vi "Fix Format String on Representation Change.vi"(8 "error in (no error)":errorcluster, 11 "Numeric Data Type in":refnum<class "Numeric Data Type.lvclass">) -> (0 "error out":errorcluster, 3 "Numeric Data Type out":refnum<class "Numeric Data Type.lvclass">)   [LabVIEW 2018, in "Numeric Data Type.lvclass"]
uses:
  Numeric Data Type.lvclass
  Numeric Data Type.lvclass/Numeric Data Type.ctl
  Numeric Format Enum.ctl
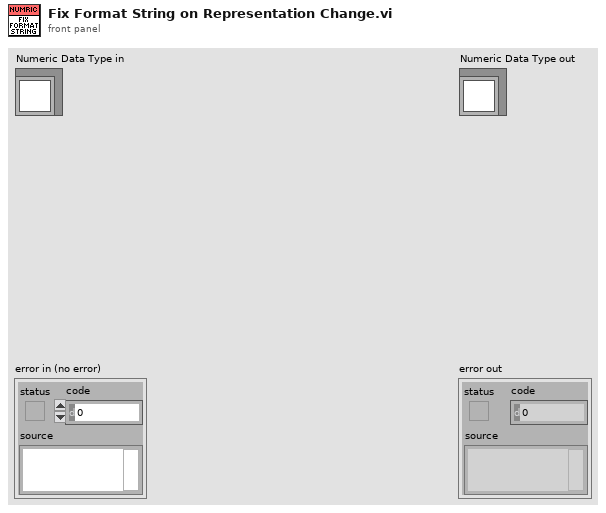
[diagram p1: front panel]
types:
  T1 = typedef "Numeric Data Type.lvclass/Numeric Format Enum.ctl" = enum16{"Floating Point Notation", "Scientific Notation", "Engineering Notation", "SI Notation", "<not used>", "Decimal", "Hexadecimal", "Octal", "Binary", "<not used 2>", "Absolute Time", "Relative Time"}
  T2 = typedef "Numeric Data Type.lvclass/Representation Enum.ctl" = enum16{"Extended (EXT)", "Double (DBL)", "Single (SGL)", "Fixed-Point (FXP)", "Quad Integer (I64)", "Long Integer (I32)", "Word Integer (I16)", "Byte Integer (I8)", "Unsigned Quad (U64)", "Unsigned Long (U32)", "Unsigned Word (U16)", "Unsigned Byte (U8)", "Complex Extended (CXT)", "Complex Double (CDB)", "Complex Single (CSG)"}
  T3 = typedef "Numeric Data Type.lvclass/Numeric Info.ctl" = cluster{"Minimum Field Width":i32, "Digits of Precision":i32, "Numeric Format":T1, "Precision Type":T4, "Hide trailing zeros":bool, "exponent":bool, "just/pad":T5, "Modifiers":string}
  T4 = typedef "Numeric Data Type.lvclass/Precision Type.ctl" = enum16{"Digits of precision", "Significant digits"}
  T5 = typedef "Numeric Data Type.lvclass/Padding.ctl" = enum16{"Pad with spaces on left", "Pad with spaces on right", "Pad with zeros on left"}
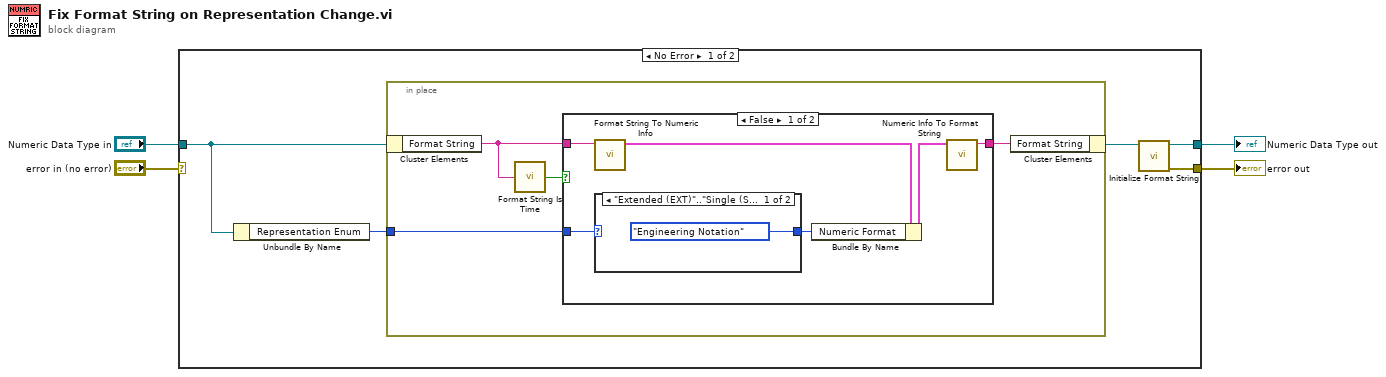
[diagram p0: block diagram]
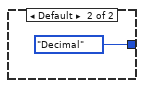
[diagram p2: hidden frame]
diagram:
  n1 = case shown="No Error" "error in (no error)" {
    selector: "error in (no error)" -> [_ w24]
    tunnel: [w5 w24] -> w3
    tunnel: [w6 w23] -> w1
    tunnel: "Numeric Data Type in" -> [w9 w23]
    frame No Error {
      n2 = Unbundle By Name(w9) -> ("Representation Enum"=w8:T2)
      n3 = in-place {
        in-place-border: w8 -> [w10]
        n4 = in-place-cluster #1(w9) -> ("Format String"=w12:string)
        n5 = call "Format String Is Time.vi"("Format String"=w12) -> ("Time?"=w13:bool)
        n6 = case shown="False" w13 {
          tunnel: w12 -> [w19 w22]
          tunnel: [w16 w22] -> w11
          tunnel: w10 -> [w14 _]
          frame False {
            n7 = call "Format String To Numeric Info.vi"("Format String"=w19) -> ("Numeric Format & Precision Info"=w18:T3)  [unwired: 10 in]
            n8 = case shown="\"Extended (EXT)\"..\"Single (SGL)\"" w14 {
              tunnel: [Numeric_Format_Enum."Engineering Notation" ("Numeric Format") Numeric_Format_Enum."Decimal" ("Numeric Format")] -> w15
              frame "Extended (EXT)".."Single (SGL)" {
              }
              frame Default {
              }
            }
            n9 = Bundle By Name(cluster=w18, "Numeric Format"=w15) -> (w17:T3)
            n10 = call "Numeric Info To Format String.vi"("Numeric Format & Precision Info"=w17) -> ("Format String"=w16:string)  [unwired: 10 in]
          }
          frame True {
          }
        }
        n11 = in-place-cluster #1("Format String"=w11) -> (w7:refnum<class "Numeric Data Type.lvclass">)
      }
      n12 = call "Initialize Format String.vi"("Numeric Data Type in"=w7) -> ("error out"=w5:errorcluster, "Numeric Data Type (dup)"=w6:refnum<class "Numeric Data Type.lvclass">)  [unwired: 9 in]
    }
    frame Error {
    }
  }
  "error out" <- w3
  "Numeric Data Type out" <- w1
